vi "gun_create.vi"(11 "Robot":T1) -> ()   [LabVIEW 2011]
uses:
  Robot Ctl.ctl
  <vilib>/Rock Robotics/SystemInterfaces/DIO/FPGA_DIOPWMChannel.ctl
  <vilib>/Rock Robotics/SystemInterfaces/DIO/FPGA_DIOChannel.ctl
  <vilib>/Rock Robotics/SystemInterfaces/AI/FPGA_AIChannel.ctl
  <vilib>/Rock Robotics/SystemInterfaces/Typedef/FPGA_TypedefAnalogModule.ctl
  <vilib>/Rock Robotics/SystemInterfaces/Typedef/FPGA_TypedefDigitalModule.ctl
  <vilib>/Rock Robotics/SystemInterfaces/DIO/FPGA_DIORelayChannel.ctl
  <vilib>/Rock Robotics/WPI/MotorControl/WPI_MotorControlOpen Victor.vi
  <vilib>/Rock Robotics/WPI/Counter/WPI_CounterDigitalInputToDigitalSource.vi
  <vilib>/Rock Robotics/WPI/Counter/WPI_CounterOpen UpDown Mode.vi
  Program Files (x86)/National Instruments/LabVIEW 2011/examples/FRC/I2C/HiTechnic Compass/Driver/HiTechnic Compass.lvlib
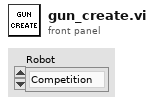
[diagram p1: front panel]
types:
  T1 = typedef "Robot Ctl.ctl" = enum16{"Competition", "Practice"}
  T2 = typedef "FPGA_DIORelayChannel.ctl" = enum8{"Relay 1", "Relay 2", "Relay 3", "Relay 4", "Relay 5", "Relay 6", "Relay 7", "Relay 8", "Invalid"}
  T3 = typedef "FPGA_TypedefDigitalModule.ctl" = enum16{"Digital Module 1", "Digital Module 2"}
  T4 = typedef "FPGA_AIChannel.ctl" = enum8{"AI 1", "AI 2", "AI 3", "AI 4", "AI 5", "AI 6", "AI 7", "AI 8", "Invalid"}
  T5 = typedef "FPGA_TypedefAnalogModule.ctl" = enum16{"Analog Module 1", "Analog Module 2"}
  T6 = typedef "FPGA_DIOPWMChannel.ctl" = enum8{"PWM 1", "PWM 2", "PWM 3", "PWM 4", "PWM 5", "PWM 6", "PWM 7", "PWM 8", "PWM 9", "PWM 10", "Invalid"}
  T7 = typedef "FPGA_DIOChannel.ctl" = enum8{"DIO 1", "DIO 2", "DIO 3", "DIO 4", "DIO 5", "DIO 6", "DIO 7", "DIO 8", "DIO 9", "DIO 10", "DIO 11", "DIO 12", "DIO 13", "DIO 14", "Invalid"}
  T8 = typedef "WPI_RelayDevRef.ctl" = cluster{"DevStatus":errorcluster, "Relay Channel":T2, "Digital Module":T3, "Relay Direction":T9}
  T9 = typedef "WPI_RelayDirection.ctl" = enum16{"Both directions", "Forward only", "Reverse only"}
  T10 = typedef "WPI_MotorControlDeviceRef.ctl" = cluster{"DeviceStatus":errorcluster, "Type":enum16{"PWM", "CAN"}, "PWM":cluster{"Digital Module":T3, "PWM Channel":T6, "DeadBand":T11}, "CAN":cluster{"Device Number":u8, "Control Mode":T12, "Semaphore":T13, "Max Vout":dbl}, "Invert":bool, "TransformRef":T14, "InvTransformRef":T14}
  T11 = typedef "WPI_PWMDeadband.ctl" = cluster{"Name":string, "maxPositivePwm":i32, "minPositivePwm":i32, "centerPwm":i32, "maxNegativePwm":i32, "minNegativePwm":i32, "angularRange":u16}
  T12 = typedef "WPI_CANJaguar_ControlMode.ctl" = enum8{"Percent VBus", "Current", "Speed", "Position", "Voltage"}
  T13 = typedef "Semaphore RefNum" = refnum<k1>
  T14 = typedef "WPI_PWMTransform_ConPane.ctl" = refnum<vi>
  T15 = typedef "WPI_AnalogChannelDevRef.ctl" = cluster{"DevStatus":errorcluster, "Analog Module":T5, "Analog Channel":T4}
  T16 = typedef "WPI_DigitalInputDevRef.ctl" = cluster{"DevStatus":errorcluster, "DIO Channel":T7, "Digital Module":T3}
  T17 = typedef "WPI_I2CDevRef.ctl" = cluster{"DevStatus":errorcluster, "Digital Module":T3, "Device Address":u8}
  T18 = typedef "FPGA_CounterEncoderSourceConvertionLVSourceType.ctl" = cluster{"DevStatus":errorcluster, "AnalogTriggerMode?":bool, "DigitalMode":cluster{"Digital Module":T3, "DIO Channel":T19}, "AnalogTriggerMode":cluster{"AnalogTriggerIndex":T20, "OutputType":T21}}
  T19 = typedef "FPGA_DIODigitalSourceChannel.ctl" = enum8{"DIO 1", "DIO 2", "DIO 3", "DIO 4", "DIO 5", "DIO 6", "DIO 7", "DIO 8", "DIO 9", "DIO 10", "DIO 11", "DIO 12", "DIO 13", "DIO 14", "Disabled"}
  T20 = typedef "FPGA_AnalogTriggerIndex.ctl" = enum8{"Trig 0", "Trig 1", "Trig 2", "Trig 3", "Trig 4", "Trig 5", "Trig 6", "Trig 7", "Invalid"}
  T21 = typedef "FPGA_AnalogTriggerOutType.ctl" = enum16{"InWindow", "TriggerState", "Rising", "Falling"}
  T22 = typedef "WPI_CounterDevRef.ctl" = cluster{"DevStatus":errorcluster, "CntIndex":T23}
  T23 = typedef "FPGA_CounterCtrSystemIndex.ctl" = enum8{"Ctr 0", "Ctr 1", "Ctr 2", "Ctr 3", "Ctr 4", "Ctr 5", "Ctr 6", "Ctr 7", "Invalid"}
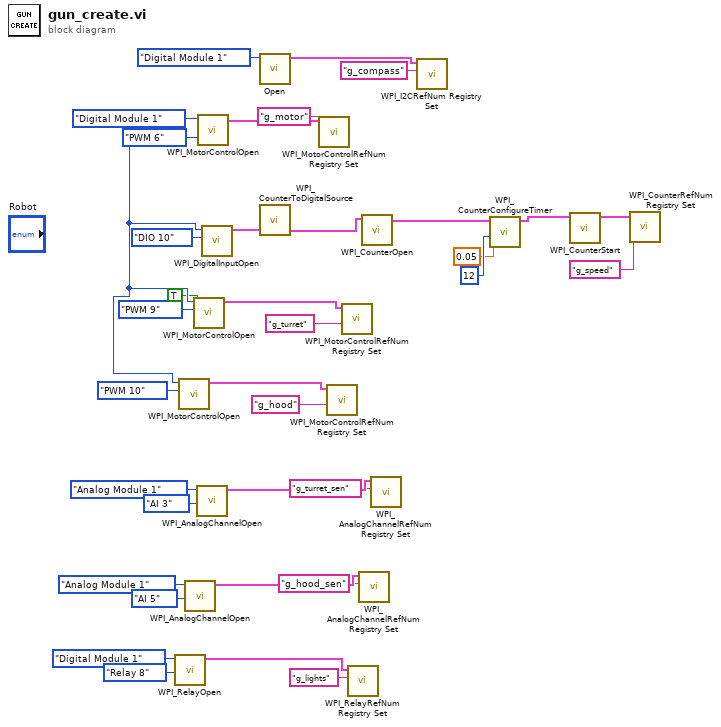
[diagram p0: block diagram]
diagram:
  w13 = FPGA_TypedefDigitalModule."Digital Module 1" ("Digital Module (Module 1)")
  n1 = call <vilib>:"WPI_RelayOpen.vi"("Relay Channel"=FPGA_DIORelayChannel."Relay 8", "Digital Module (Module 1)"=FPGA_TypedefDigitalModule."Digital Module 1") -> ("RelayDevRef"=w3:T8)  [unwired: 8 in, 1 out]
  n2 = call-poly <vilib>:"WPI_MotorControlOpen.vi"("PWM Channel"=FPGA_DIOPWMChannel."PWM 10", "Digital Module (Module 1)"=w13) -> ("MotorControlDeviceRef"=w15:T10)  [unwired: 8 in, 1 out]
  n3 = call <vilib>:"WPI_AnalogChannelOpen.vi"("Analog Channel"=FPGA_AIChannel."AI 5", "Analog Module (Module 1)"=FPGA_TypedefAnalogModule."Analog Module 1") -> ("AIDeviceRef"=w11:T15)  [unwired: 8 in, 1 out]
  n4 = call-poly <vilib>:"WPI_MotorControlOpen.vi"("Eliminate Deadband"=TRUE, "PWM Channel"=FPGA_DIOPWMChannel."PWM 9", "Digital Module (Module 1)"=w13) -> ("MotorControlDeviceRef"=w22:T10)  [unwired: 7 in, 1 out]
  n5 = call <vilib>:"WPI_AnalogChannelOpen.vi"("Analog Channel"=FPGA_AIChannel."AI 3", "Analog Module (Module 1)"=FPGA_TypedefAnalogModule."Analog Module 1") -> ("AIDeviceRef"=w19:T15)  [unwired: 8 in, 1 out]
  n6 = call-poly <vilib>:"WPI_MotorControlOpen.vi"("PWM Channel"=FPGA_DIOPWMChannel."PWM 6", "Digital Module (Module 1)"=w13) -> ("MotorControlDeviceRef"=w34:T10)  [unwired: 8 in, 1 out]
  n7 = call <vilib>:"WPI_DigitalInputOpen.vi"("DIO Channel"=FPGA_DIOChannel."DIO 10", "Digital Module (Module 1)"=w13) -> ("DigitalInputDevRef"=w25:T16)  [unwired: 8 in, 1 out]
  n8 = call "Open.vi"("DigitalModule"=FPGA_TypedefDigitalModule."Digital Module 1") -> ("I2CDevRef"=w8:T17)  [unwired: 1 in, 9 out]
  n9 = call-poly <vilib>:"WPI_CounterToDigitalSource.vi"("DigitalInputDevRef"=w25) -> ("Digital Source"=w28:T18)  [unwired: 6 in]
  n10 = call <vilib>:"WPI_MotorControlRefNum Registry Set.vi"("refnum name"="g_motor", "MotorControlDevRef"=w34) -> ()  [unwired: 8 in, 2 out]
  n11 = call <vilib>:"WPI_MotorControlRefNum Registry Set.vi"("refnum name"="g_hood", "MotorControlDevRef"=w15) -> ()  [unwired: 8 in, 2 out]
  n12 = call <vilib>:"WPI_MotorControlRefNum Registry Set.vi"("refnum name"="g_turret", "MotorControlDevRef"=w22) -> ()  [unwired: 8 in, 2 out]
  n13 = call <vilib>:"WPI_RelayRefNum Registry Set.vi"("refnum name"="g_lights", "RelayDevRef"=w3) -> ()  [unwired: 8 in, 2 out]
  n14 = call <vilib>:"WPI_AnalogChannelRefNum Registry Set.vi"("refnum name"="g_hood_sen", "AIDeviceRef"=w11) -> ()  [unwired: 8 in, 2 out]
  n15 = call-poly <vilib>:"WPI_CounterOpen.vi"("Up Source"=w28) -> ("CounterDevRef"=w29:T22)  [unwired: 9 in, 1 out]
  n16 = call <vilib>:"WPI_AnalogChannelRefNum Registry Set.vi"("refnum name"="g_turret_sen", "AIDeviceRef"=w19) -> ()  [unwired: 8 in, 2 out]
  n17 = call <vilib>:"WPI_I2CRefNum Registry Set.vi"("refnum name"="g_compass", "I2CDevRef"=w8) -> ()  [unwired: 8 in, 2 out]
  n18 = call <vilib>:"WPI_CounterConfigureTimer.vi"("Number Samples to Average"=u8 12, "MaxPeriod (sec)"=0.05, "CounterDevRef in"=w29) -> ("CounterDevRef out"=w30:T22)  [unwired: 7 in, 1 out]
  n19 = call <vilib>:"WPI_CounterStart.vi"("CounterDevRef in"=w30) -> ("CounterDevRef out"=w31:T22)  [unwired: 9 in, 1 out]
  n20 = call <vilib>:"WPI_CounterRefNum Registry Set.vi"("refnum name"="g_speed", "CounterDevRef"=w31) -> ()  [unwired: 8 in, 2 out]
